vi "HighpassPeak-Peak.vi"(8 "error in (no error)":errorcluster, 9 "Highpass Filter State":T1 {"Filter State" format="%.2f"; "IIR Filter Cluster"."Forward Coefficients" format="%.2f"; "IIR Filter Cluster"."Reverse Coefficients" format="%.2f"}, 10 "highpass cutoff":dbl format="%#_13g", 11 "input signal":waveform(sgl)) -> (0 "error out":errorcluster, 1 "Highpass Filter State out":T1 {"Filter State" format="%.2f"; "IIR Filter Cluster"."Forward Coefficients" format="%.2f"; "IIR Filter Cluster"."Reverse Coefficients" format="%.2f"}, 2 "pk-pk":dbl, 5 "valid":bool)   [LabVIEW 2017, in "VibrationAnalysisFunctions.lvlib"]
uses:
  <vilib>/addons/InsightCM/Utilities/Analysis/Vibration/VibrationAnalysisFunctions.lvlib
  <vilib>/addons/InsightCM/Utilities/Analysis/Vibration/controls/HighPassFilterState.ctl
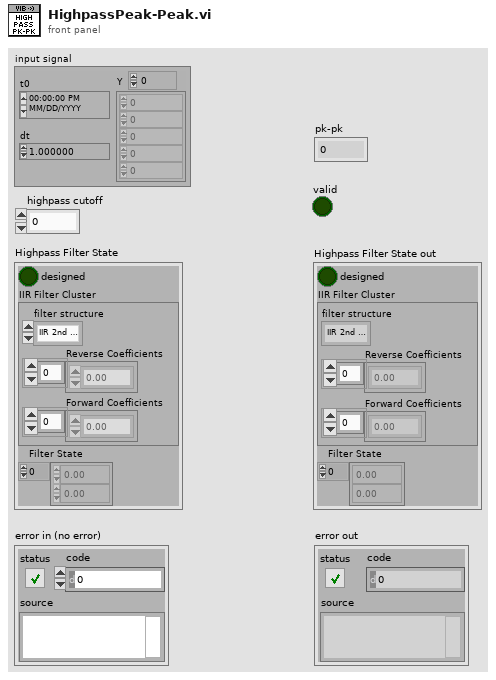
[diagram p1: front panel]
types:
  T1 = typedef "VibrationAnalysisFunctions.lvlib/HighPassFilterState.ctl" = cluster{"designed":bool, "IIR Filter Cluster":cluster{"filter structure":enum32{"IIR 2nd Order", "IIR 4th Order"}, "Reverse Coefficients":dbl[], "Forward Coefficients":dbl[]}, "Filter State":dbl[]}
  T2 = cluster{"filter structure":enum32{"IIR 2nd Order", "IIR 4th Order"}, "Reverse Coefficients":dbl[], "Forward Coefficients":dbl[]}
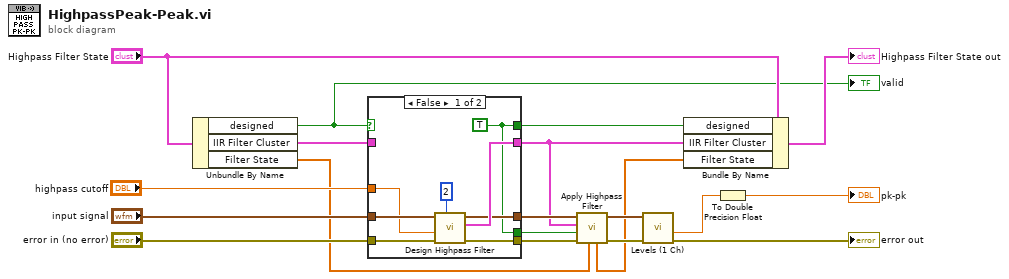
[diagram p0: block diagram]
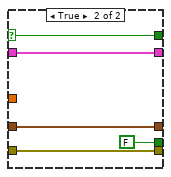
[diagram p2: hidden frame]
diagram:
  n1 = Unbundle By Name("Highpass Filter State") -> ("designed"=w2:bool, "IIR Filter Cluster"=w10:T2, "Filter State"=w9:dbl[])
  "valid" <- w2
  n2 = case shown="False" w2 {
    selector: w2 -> [_ w28]
    tunnel: [w27 w32] -> w6
    tunnel: [w26 w31] -> w19
    tunnel: "error in (no error)" -> [w25 w30]
    tunnel: [w24 w30] -> w17
    tunnel: "input signal" -> [w22 w31]
    tunnel: w10 -> [_ w32]
    tunnel: [w20 FALSE] -> w12
    tunnel: "highpass cutoff" -> [w21 _]
    tunnel: [w20 w28] -> w7
    frame False {
      w20 = TRUE
      n3 = call <vilib>:"Design Highpass Filter.vi"("highpass filter order"=2, "error in (no error)"=w25, "highpass cutoff frequency"=w21, "input signal"=w22) -> ("error out"=w24:errorcluster, "IIR Filter Cluster"=w27:T2, "dup signal"=w26:waveform(sgl))  [unwired: 5 in]
    }
    frame True {
    }
  }
  n4 = call <vilib>:"Apply Highpass Filter.vi"("Initial Filter State"=w9, "error in (no error)"=w17, "init/cont (init:F)"=w12, "filter coefficients"=w6, "signal [V]"=w19) -> ("error out"=w15:errorcluster, "filtered signal [EU]"=w14:waveform(sgl), "Final Filter State"=w5:dbl[])  [unwired: 4 in]
  n5 = call <vilib>:"Levels (1 Ch).vi"("error in (no error)"=w15, "Waveform"=w14) -> ("error out"=→"error out":errorcluster, "Pk-Pk"=w1:sgl)  [unwired: 4 in, 4 out]
  n6 = Bundle By Name(cluster="Highpass Filter State", "designed"=w7, "IIR Filter Cluster"=w6, "Filter State"=w5) -> (→"Highpass Filter State out":T1)
  n7 = To Double Precision Float(number=w1) -> (double precision float=→"pk-pk":dbl)
